vi "CH_LM Test File Manager.vi"() -> ()   [LabVIEW 2012, in "CH_LM.lvlib"]
doc: "This example VI can be used to browse and manipulated the directories and files on the remote LabMax device.\n\n<B>Note:</B> Since directories are not yet returned from the catalog query this VI is of limited use. Further developmentof this is deferred until this feature becomes available."
uses:
  CH_LM.lvlib
  CH_LM App.lvlib
  CH_LM/CH_LM BaudRates.ctl
  CH_LM/CH_LM Parity.ctl
  CH_LM/CH_LM SerialConfiguration.ctl
panel:
  in  "Serial Configuration\n(19200,N,8,1)":T1={"Baud Rate"=19200, "Parity"=0, "Data Bits"=8, "Stop Bits"=1} {"Parity" items=["None", "Odd", "Even"]; "Baud Rate" items=["9600"=9600, "19200"=19200, "38400"=38400, "57600"=57600, "115200"=115200]}
  out "Tree.DC.Value":string
  out "Tree.MD.Value":string
  out "Tree.NewVal":string
  in  "Update":bool
  out "Lock timed out":bool
  in  "Tree":string(tree)
  out "number of files found":i32
  in  "pattern":string=".?"
  in  "Path to start the search":string="\\loc"
  in  "Reset":bool
  out "error out":errorcluster
  in  "stop":bool
  out "timed out?":bool
  in  "Address":i32=1
  in  "Serial Number":string
  in  "Reset? (F: No)":bool
  in  "ID Query? (T: Yes)":bool
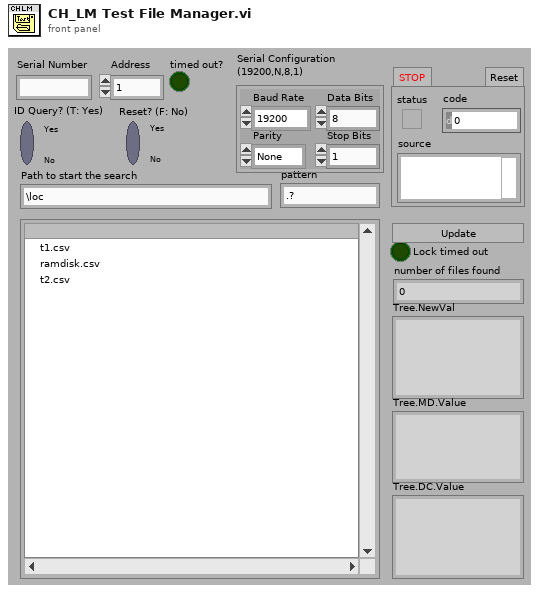
[diagram p1: front panel]
types:
  T1 = typedef "CH_LM.lvlib/CH_LM SerialConfiguration.ctl" = cluster{"Baud Rate":T2, "Parity":T3, "Data Bits":u16, "Stop Bits":u16}
  T2 = typedef "CH_LM.lvlib/CH_LM BaudRates.ctl" = u32
  T3 = typedef "CH_LM.lvlib/CH_LM Parity.ctl" = u16
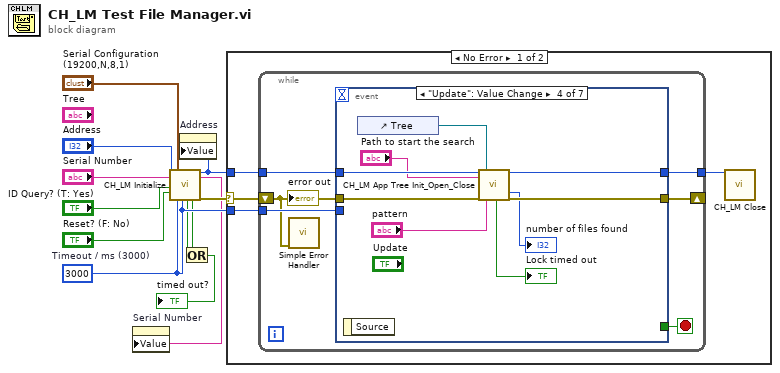
[diagram p0: block diagram]
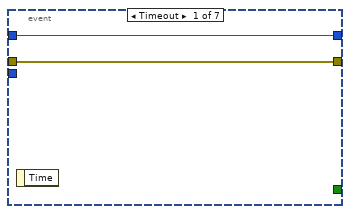
[diagram p2: hidden frame]
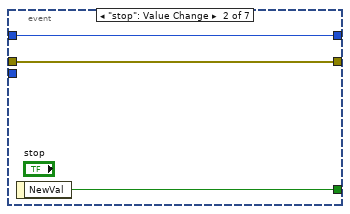
[diagram p3: hidden frame]
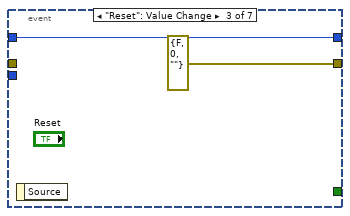
[diagram p4: hidden frame]
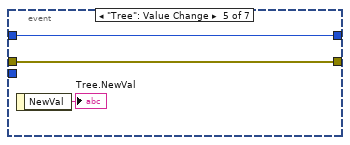
[diagram p5: hidden frame]
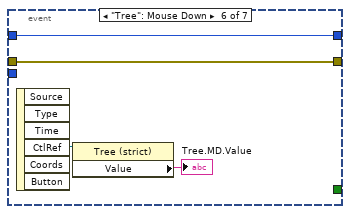
[diagram p6: hidden frame]
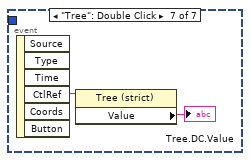
[diagram p7: hidden frame]
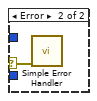
[diagram p8: hidden frame]
diagram:
  w9 = 3000  # Timeout / ms (3000)
  n1 = call "CH_LM Initialize.vi"("Address"="Address", "Serial Number"="Serial Number", "ID Query (True)"="ID Query? (T: Yes)", "Reset (False)"="Reset? (F: No)", "Serial Configuration\n(19200,N,8,1)"="Serial Configuration\n(19200,N,8,1)", "Timeout / ms (3000)"=w9, "Lock Timeout / ms (1000)"=w9) -> ("Lock timed out"=w8:bool, "timed out?"=w7:bool, "Meter Index"=w3:i32, "Serial Number"=w2:string, "error out"=w10:errorcluster)  [unwired: 1 in, 7 out]
  n2 = property on="Serial Number" class="Str"("Value"=w2) -> ()  [unwired: 2 in, 2 out]
  n3 = property on="Address" class="DigNum (strict)"("Value"=w3) -> ()  [unwired: 2 in, 2 out]
  n4 = Or(x=w7, y=w8) -> (x .or. y?=→"timed out?":bool)
  n5 = case shown="No Error" w10 {
    selector: w10 -> [w13 w48]
    tunnel: w3 -> [w14 _]
    tunnel: w9 -> [w15 _]
    frame No Error {
      n6 = while {
        tunnel: w14 -> [w22]
        tunnel: [w21] -> w16
        shift-right: [w20] -> _
        shift-left: w13 -> [w17]
        tunnel: w15 -> [w19]
        stop <- w18 stop-if-true
        n7 = call <vilib>:"Simple Error Handler.vi"("error in (no error)"=w17) -> ()  [unwired: 1 in, 8 out]
        n8 = event shown="[3] \"Update\": Value Change" {
          selector: _ -> [_ _ _ _ _ _ _]
          dyn-events: _ -> [_ _ _ _ _ _ _]
          timeout: _ -> [_ _ _ _ _ _ _]
          tunnel: [_ w27 _ _ _ _ _] -> w18
          tunnel: w22 -> [w23 w26 w28 w37 w40 w43 _]
          tunnel: w17 -> [w24 w25 _ w35 w39 w42 _]
          tunnel: [w23 w26 w28 w36 w40 w43 _] -> w21
          tunnel: [w24 w25 errorcluster {"status"=FALSE, "code"=0, "source"=""} ("error out") w34 w39 w42 _] -> w20
          tunnel: w19 -> [_ _ _ _ _ _ _]
          event Timeout {
            n9 = event-data() -> ()  [unwired: 2 out]
          }
          event "stop": Value Change {
            n10 = event-data() -> ("NewVal"=w27:bool)  [unwired: 1 out]
          }
          event "Reset": Value Change {
            n11 = event-data() -> ()  [unwired: 2 out]
          }
          event "Update": Value Change {
            n12 = event-data() -> ()  [unwired: 2 out]
            n13 = control-ref of="Tree"() -> (w38:refnum<vi>)
            n14 = call "CH_LM App Tree Init_Open_Close.vi"("Meter Index"=w37, "path to start the search"="Path to start the search", "error in"=w35, "Tree In"=w38, "pattern"="pattern") -> ("Lock timed out"=→"Lock timed out":bool, "Meter Index"=w36:i32, "Number of files found"=→"number of files found":i32, "error out"=w34:errorcluster)  [unwired: 2 in, 9 out]
          }
          event "Tree": Value Change {
            n15 = event-data() -> ("NewVal"=→"Tree.NewVal":string)  [unwired: 1 out]
          }
          event "Tree": Mouse Down {
            n16 = event-data() -> ("CtlRef"=w45:refnum<vi>)  [unwired: 6 out]
            n17 = property class="Tree (strict)"(reference=w45) -> ("Value"=→"Tree.MD.Value":string)  [unwired: 1 in, 2 out]
          }
          event "Tree": Double Click {
            n18 = event-data() -> ("CtlRef"=w47:refnum<vi>)  [unwired: 6 out]
            n19 = property class="Tree (strict)"(reference=w47) -> ("Value"=→"Tree.DC.Value":string)  [unwired: 1 in, 2 out]
          }
        }
        "error out" <- w17
      }
      n20 = call "CH_LM Close.vi"("Meter Index"=w16) -> ()  [unwired: 1 in, 18 out]
    }
    frame Error {
      n21 = call <vilib>:"Simple Error Handler.vi"("error in (no error)"=w48) -> ()  [unwired: 1 in, 8 out]
    }
  }
